vi "pcfs_move_axis.vi"(8 "error in (no error)":errorcluster, 9 "Speed":dbl, 10 "position":dbl, 11 "pcfs in":refnum<class "pcfs.lvclass">) -> (0 "error out":errorcluster, 3 "pcfs out":refnum<class "pcfs.lvclass">)   [LabVIEW 2015, in "pcfs.lvclass"]
uses:
  pcfs.lvclass
  pcfs.lvclass/pcfs.ctl
  Stage Class/Stage.lvclass
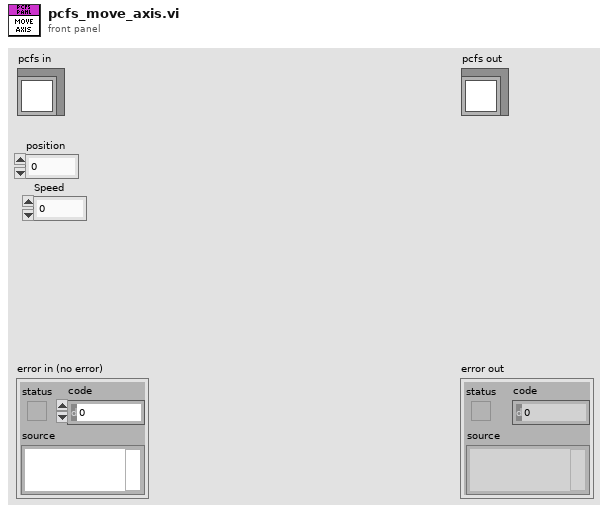
[diagram p1: front panel]
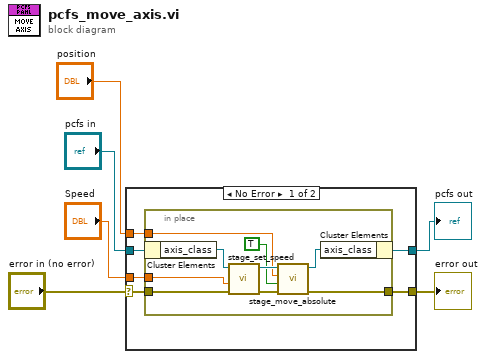
[diagram p0: block diagram]
diagram:
  n1 = case shown="No Error" "error in (no error)" {
    selector: "error in (no error)" -> [w10 w23]
    tunnel: [w9 w23] -> w5
    tunnel: [w7 w22] -> w3
    tunnel: "pcfs in" -> [w12 w22]
    tunnel: "Speed" -> [w11 _]
    tunnel: "position" -> [w8 _]
    frame No Error {
      n2 = in-place {
        in-place-border: w11 -> [w17]
        in-place-border: w10 -> [w16]
        in-place-border: [w15] -> w9
        in-place-border: w8 -> [w13]
        n3 = in-place-cluster #1(w12) -> ("axis_class"=w18:refnum<class "Stage.lvclass">)
        n4 = call-dynamic "stage_set_speed.vi"("error in (no error)"=w16, "Speed"=w17, "Stage in"=w18) -> ("error out"=w21:errorcluster, "Stage out"=w20:refnum<class "Stage.lvclass">)  [unwired: 7 in]
        n5 = call-dynamic "stage_move_absolute.vi"("error in (no error)"=w21, "wait_for_done"=TRUE, "Position"=w13, "Stage in"=w20) -> ("error out"=w15:errorcluster, "Stage out"=w14:refnum<class "Stage.lvclass">)  [unwired: 6 in]
        n6 = in-place-cluster #1("axis_class"=w14) -> (w7:refnum<class "pcfs.lvclass">)
      }
    }
    frame Error {
    }
  }
  "error out" <- w5
  "pcfs out" <- w3
